vi "Simple Reader.vi"(8 "error in (no error)":errorcluster, 11 "PLL reader in":refnum<class "PLL reader.lvclass">) -> (0 "error out":errorcluster, 2 "Signals":dbl[](array[numeric]), 3 "PLL reader out":refnum<class "PLL reader.lvclass">)   [LabVIEW 2018, in "PLL reader.lvclass"]
uses:
  PLL reader.lvclass
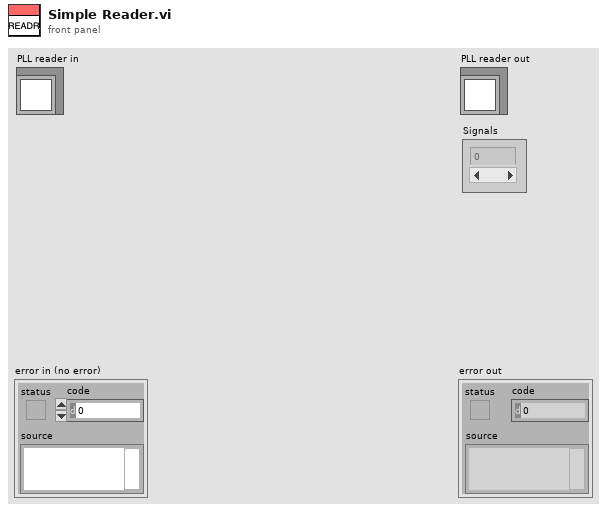
[diagram p1: front panel]
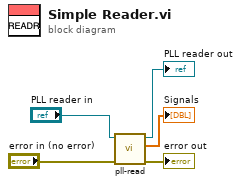
[diagram p0: block diagram]
diagram:
  n1 = call "pll-read.vi"("error in (no error)"="error in (no error)", "PLL reader.lvclass"="PLL reader in") -> ("error out"=→"error out":errorcluster, "Result"=→"Signals":dbl[], "PLL reader.lvclass Out"=→"PLL reader out":refnum<class "PLL reader.lvclass">)  [unwired: 7 in]
